vi "Temperature Log.vi"() -> ()   [LabVIEW 2010]
doc: "This VI is a solution to an exercise in the LabVIEW Core I course.\n\nThis VI acquires temperature values every 500 ms and also takes a running average of the last three temperature measurements and displays both the raw data and the running average in the strip chart."
panel:
  out "Temperature History":cluster{dbl, "Temperature":dbl}(graph)
  in  "Power":bool=TRUE
  # "ON\n\nOFF"
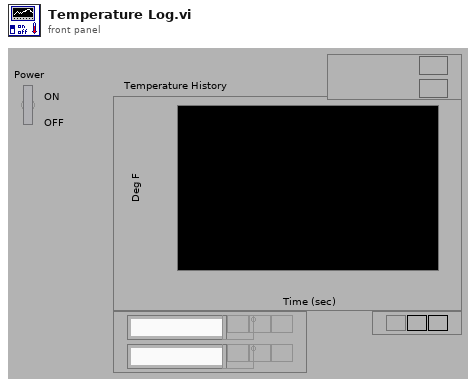
[diagram p1: front panel]
types:
  T1 = enum16{"open", "replace", "create", "open or create", "replace or create", "replace or create with confirmation"}
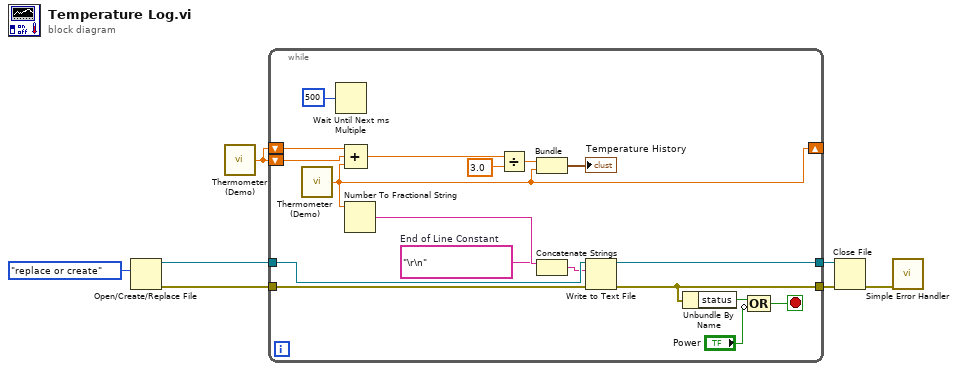
[diagram p0: block diagram]
diagram:
  n1 = Open/Create/Replace File(operation (0:open)=T1."replace or create") -> (refnum out=w7:refnum<file>, error out=w5:errorcluster)  [unwired: 1 in, 5 out]
  n2 = call "Thermometer (Demo).vi"() -> ("Temperature"=w1:dbl)  [unwired: 1 in]
  n3 = while {
    shift-left: w1 -> [w22]
    shift-left: w1 -> [w23]
    shift-right: [w9] -> _
    tunnel: w7 -> [w18]
    tunnel: [w17] -> w6
    tunnel: w5 -> [w16]
    tunnel: [w12] -> w4
    stop <- w11 stop-if-true
    w14 = "\r\n"  # End of Line Constant
    n4 = call "Thermometer (Demo).vi"() -> ("Temperature"=w9:dbl)  [unwired: 1 in]
    n5 = Wait Until Next ms Multiple(millisecond multiple=u32 500) -> ()  [unwired: 1 out]
    n6 = Compound Arithmetic op=ADD(w23, w22, w9) -> (w21:dbl)
    n7 = Number To Fractional String(number=w9) -> (F-format string=w15:string)  [unwired: 3 out]
    n8 = Divide(x=w21, y=3.0 ("number: 0 to 1")) -> (x/y=w20:dbl)
    n9 = Bundle(w20, "Temperature"=w9) -> (→"Temperature History":cluster{dbl, "Temperature":dbl})  [unwired: 1 out]
    n10 = Concatenate Strings(w15, w14) -> (w13:string)
    n11 = Write to Text File(file (use dialog)=w18, text=w13, error in=w16) -> (refnum out=w17:refnum<file>, error out=w12:errorcluster)  [unwired: 2 out]
    n12 = Unbundle By Name(w12) -> ("status"=w8:bool)
    n13 = Compound Arithmetic op=OR(w8, invert "Power") -> (w11:bool)
  }
  n14 = Close File(refnum=w6, error in=w4) -> (error out=w3:errorcluster)  [unwired: 1 out]
  n15 = call <vilib>:"Simple Error Handler.vi"("error in (no error)"=w3) -> ()  [unwired: 1 in, 8 out]
